vi "Exit.vi"(8 "error in (no error)":errorcluster, 10 "Data":variant, 11 "PID Loop in":refnum<class "PID Loop.lvclass">) -> (0 "error out":errorcluster, 3 "PID Loop out":refnum<class "PID Loop.lvclass">)   [LabVIEW 2024, in "PID Loop.lvlib" / "PID Loop.lvclass"]
uses:
  PID Loop.lvclass
  PID Loop.lvclass/PID Loop.ctl
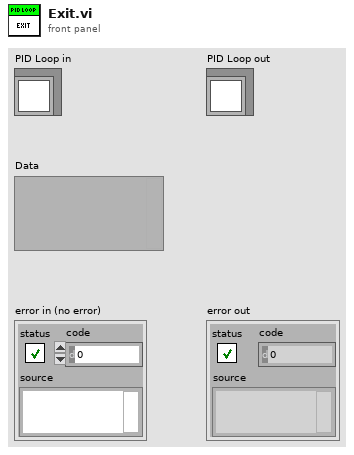
[diagram p1: front panel]
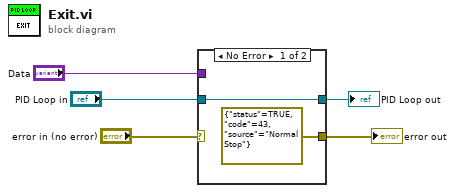
[diagram p0: block diagram]
diagram:
  n1 = case shown="No Error" "error in (no error)" {
    selector: "error in (no error)" -> [_ w9]
    tunnel: [errorcluster {"status"=TRUE, "code"=43, "source"="Normal Stop"} ("error IO") w9] -> w4
    tunnel: [w7 w8] -> w2
    tunnel: "PID Loop in" -> [w7 w8]
    tunnel: "Data" -> [_ _]
    frame No Error {
    }
    frame Error {
    }
  }
  "error out" <- w4
  "PID Loop out" <- w2
